vi "RM.initDatabase.vi"(8 "error in":errorcluster) -> (0 "error out":errorcluster, 3 "reservation DB out":variant)   [LabVIEW 2016, in "FPGA Resource Manager.lvlib"]
uses:
  FPGA Resource Manager.lvlib
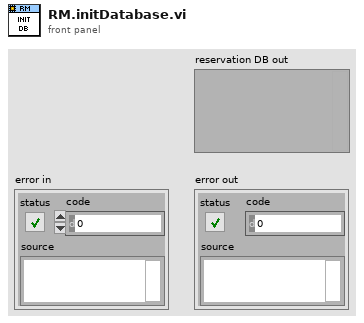
[diagram p1: front panel]
types:
  T1 = typedef "FPGA Resource Manager.lvlib/RM.resourceType.ctl" = enum16{"Scalar Input", "Scalar Output", "Waveform Input", "Waveform Output"}
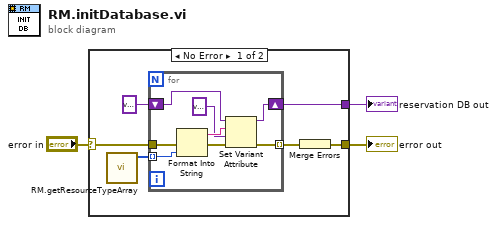
[diagram p0: block diagram]
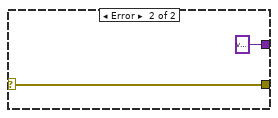
[diagram p2: hidden frame]
diagram:
  n1 = case shown="No Error" "error in" {
    selector: "error in" -> [w7 w18]
    tunnel: [w8 variant] -> w3
    tunnel: [w5 w18] -> w2
    frame No Error {
      n2 = call "RM.getResourceTypeArray.vi"() -> ("Array"=w4:T1[])  [unwired: 11 in]
      n3 = for {
        shift-right: [w12] -> w8
        shift-left: variant -> [w13]
        tunnel: w4 -> [w14] mode=indexing
        tunnel: w7 -> [w11]
        tunnel: [w10] -> w6 mode=indexing
        n4 = Format Into String(error in=w11, w14) -> (resulting string=w16:string, error out=w17:errorcluster)  [unwired: 2 in]
        n5 = Set Variant Attribute(Variant=w13, name=w16, value=variant, error in=w17) -> (Variant out=w12:variant, error out=w10:errorcluster)  [unwired: 1 out]
      }
      n6 = Merge Errors(w6) -> (w5:errorcluster)
    }
    frame Error {
    }
  }
  "reservation DB out" <- w3
  "error out" <- w2
